vi "Query Arb Waveform Capabilities [ARB].vi"(8 "error in (no error)":errorcluster, 11 "CS++Fgen in":refnum<class "CS++Fgen.lvclass">) -> (0 "error out":errorcluster, 1 "waveform quantum":i32, 2 "max number of waveforms":i32, 3 "CS++Fgen out":refnum<class "CS++Fgen.lvclass">, 4 "max waveform size":i32, 6 "min waveform size":i32)   [LabVIEW 2016, in "CS++Fgen.lvlib" / "CS++Fgen.lvclass"]
doc: "This VI returns the properties of the function generator that are related to creating arbitrary waveforms. These properties are the maximum number of waveforms, waveform quantum, minimum waveform size, and maximum waveform size.\n\nNotes:\n\n(1) This VI is part of the IviFgenArbWfm [ARB] extension group."
uses:
  CS++Fgen.lvclass
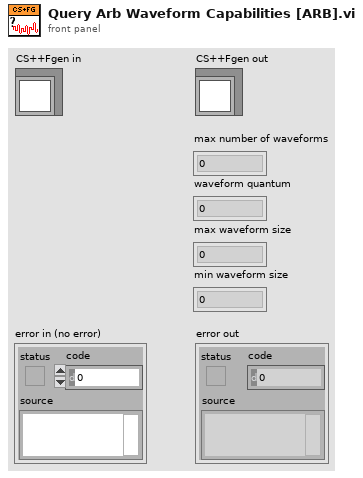
[diagram p1: front panel]
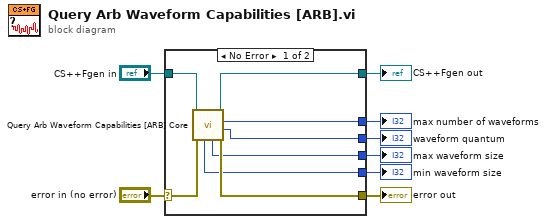
[diagram p0: block diagram]
diagram:
  n1 = case shown="No Error" "error in (no error)" {
    selector: "error in (no error)" -> [w16 w18]
    tunnel: [w15 w18] -> w7
    tunnel: [w13 w17] -> w5
    tunnel: "CS++Fgen in" -> [w14 w17]
    tunnel: [w12 _] -> w4
    tunnel: [w11 _] -> w3
    tunnel: [w10 _] -> w2
    tunnel: [w9 _] -> w1
    frame No Error {
      n2 = call-dynamic "Query Arb Waveform Capabilities [ARB] Core.vi"("error in (no error)"=w16, "CS++Fgen in"=w14) -> ("error out"=w15:errorcluster, "waveform quantum"=w11:i32, "max number of waveforms"=w12:i32, "CS++Fgen out"=w13:refnum<class "CS++Fgen.lvclass">, "max waveform size"=w10:i32, "min waveform size"=w9:i32)  [unwired: 4 in]
    }
    frame Error {
    }
  }
  "error out" <- w7
  "CS++Fgen out" <- w5
  "max number of waveforms" <- w4
  "waveform quantum" <- w3
  "max waveform size" <- w2
  "min waveform size" <- w1
